vi "GEA2 Initialize Multiple Devices.vi"(0 "Source Addresses":u8[](array[numeric]) format="%.0x", 11 "error in":errorcluster) -> (4 "Array of GEA2 References Out":refnum<k24>[](array[refnum]), 8 "Board IDs":string[](array[string]), 15 "error out":errorcluster)   [LabVIEW 2016, in "GEA2_Toolkit.lvlib"]
doc: "This VI uses .NET DLLs to initialize a GEA2 connection over USB to multiple devices. The output is an array of references to the newly opened GEA2 connections."
uses:
  library/GEA2_Toolkit.lvlib
  C:/Users/220038920/Desktop/GEA3 Toolkit/GEA3 DLL Source/GeaCommunication.dll
  GEA3 DLL Source/GeaCommunication.dll
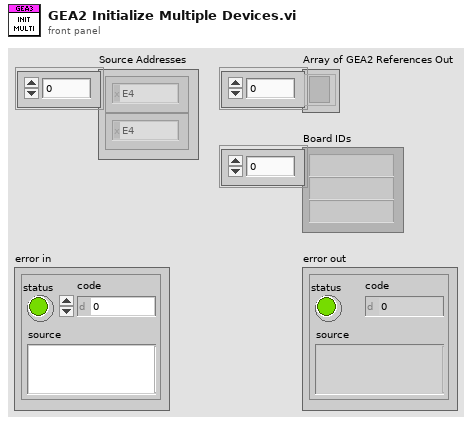
[diagram p1: front panel]
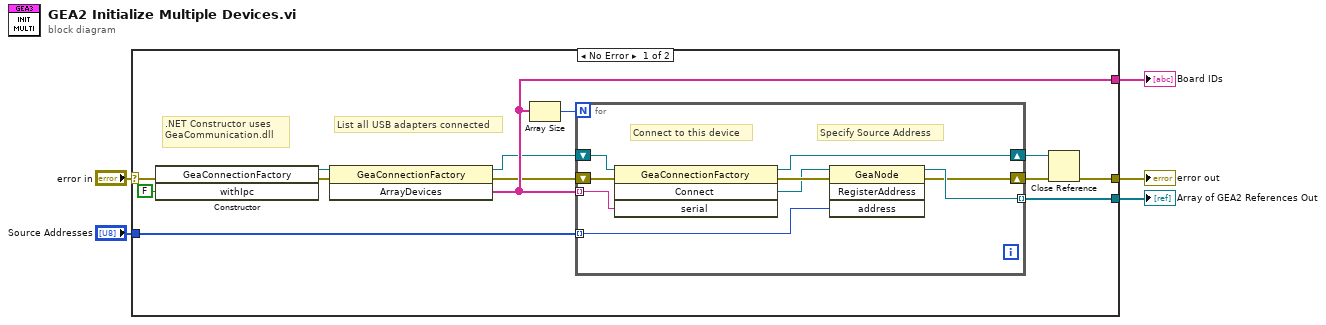
[diagram p0: block diagram]
diagram:
  n1 = case shown="No Error" "error in" {
    selector: "error in" -> [w11 w28]
    tunnel: [w13 w28] -> w5
    tunnel: [w14 _] -> w1
    tunnel: "Source Addresses" -> [w18 _]
    tunnel: [w10 _] -> w2
    frame No Error {
      # "List all USB adapters connected"
      # ".NET Constructor uses\nGeaCommunication.dll"
      n2 = constructor class="GeaConnectionFactory"(error in=w11, "withIpc"=FALSE) -> (reference out=w12:refnum<k24>, error out=w7:errorcluster)  [unwired: 2 in, 2 out]
      n3 = invoke class="GeaConnectionFactory" method="ArrayDevices"(reference=w12, error in=w7) -> (reference out=w8:refnum<k24>, error out=w9:errorcluster, "ArrayDevices"=w10:string[])  [unwired: 1 in]
      n4 = Array Size(array=w10) -> (size(s)=w17:i32)
      n5 = for {
        N: w17 -> [_]
        tunnel: [w26] -> w14 mode=indexing
        shift-right: [w23] -> w15
        shift-left: w8 -> [w24]
        shift-right: [w22] -> w16
        shift-left: w9 -> [w19]
        tunnel: w18 -> [w21] mode=indexing
        tunnel: w10 -> [w20] mode=indexing
        # "Specify Source Address"
        # "Connect to this device"
        n6 = invoke class="GeaConnectionFactory" method="Connect"(reference=w24, error in=w19, "serial"=w20) -> (reference out=w23:refnum<k24>, error out=w27:errorcluster, "Connect"=w25:refnum<k24>)  [unwired: 1 in, 1 out]
        n7 = invoke class="GeaNode" method="RegisterAddress"(reference=w25, error in=w27, "address"=w21) -> (reference out=w26:refnum<k24>, error out=w22:errorcluster)  [unwired: 1 in, 2 out]
      }
      n8 = Close Reference(reference=w15, error in (no error)=w16) -> (error out=w13:errorcluster)
    }
    frame Error {
    }
  }
  "error out" <- w5
  "Board IDs" <- w2
  "Array of GEA2 References Out" <- w1
